vi "MeasureRMS.vi"() -> ()   [LabVIEW 2015]
uses:
  <vilib>/Analysis/5stat.llb/RMS (DBL).vi
  <vilib>/Analysis/NI_AALPro.lvlib
panel:
  out "rms value":dbl format="%0.2f"
  in  "# of Samples":i32
  in  "Sampling Rate (Hz)":i32
  out "Waveform Graph":dynamicdata(graph)
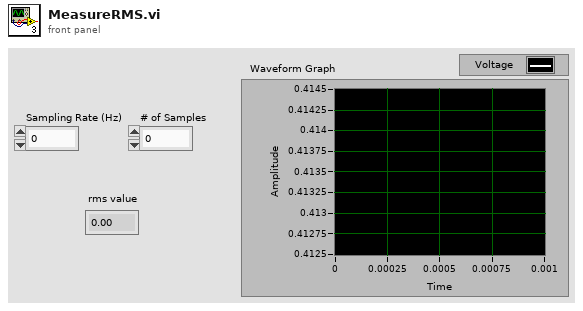
[diagram p1: front panel]
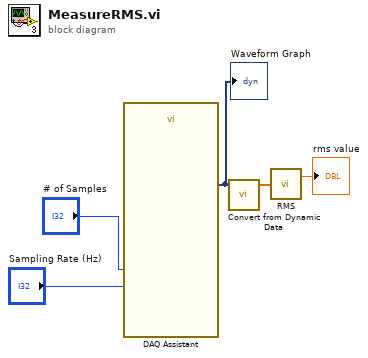
[diagram p0: block diagram]
diagram:
  n1 = call "DAQ Assistant"("rate"="Sampling Rate (Hz)", "number of samples"="# of Samples") -> ("data"=w5:dynamicdata)  [unwired: 15 in, 2 out]
  "Waveform Graph" <- w5
  n2 = call "Convert from Dynamic Data"("Dynamic Data Type"=w5) -> ("Array"=w4:dbl[])  [unwired: 3 in]
  n3 = call-poly <vilib>:"RMS.vi"("X"=w4) -> ("rms value"=→"rms value":dbl)  [unwired: 1 out]
